vi "sawtooth.vi"(9 "cycles":u32=1 min=1, 10 "samples":u32=128, 11 "amplitude in":dbl=1.0 format="%0.2f") -> (3 "sawtooth signal":dbl[](array[numeric]))   [LabVIEW 2010]
uses:
  <vilib>/Analysis/NI_AALBase.lvlib
panel:
  out "waveform":dbl[](graph)
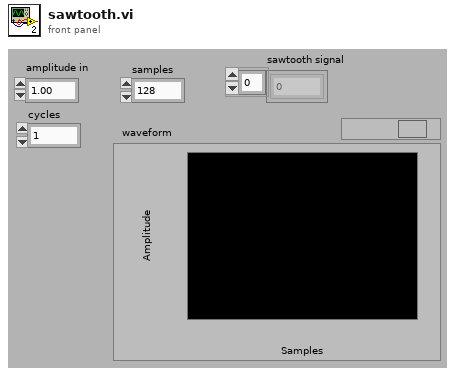
[diagram p1: front panel]
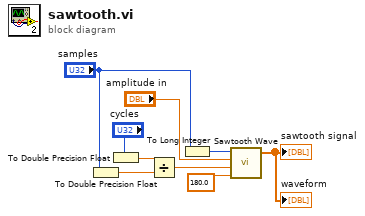
[diagram p0: block diagram]
diagram:
  n1 = To Double Precision Float(number="samples") -> (double precision float=w8:dbl)
  n2 = To Double Precision Float(number="cycles") -> (double precision float=w4:dbl)
  n3 = Divide(x=w4, y=w8) -> (x/y=w6:dbl)
  n4 = To Long Integer(number="samples") -> (32bit integer=w1:i32)
  n5 = call <vilib>:"Sawtooth Wave.vi"("samples"=w1, "amplitude"="amplitude in", "frequency"=w6, "phase in"=180.0) -> ("sawtooth wave"=→"sawtooth signal" →"waveform":dbl[])  [unwired: 1 in, 2 out]
